vi "Motor-Pega-Vel_Acc.vi"(4 "error out":errorcluster, 7 "MG17Motor in":refnum<k7>) -> (0 "error out 2":errorcluster, 1 "pfAccn":sgl, 2 "pfMaxVel":sgl, 3 "MG17Motor out":refnum<k7>)   [LabVIEW 2014]
doc: "This VI get Velocity and Acceleration of Motor\n\nAndré Romero - 2023\nandretec@ifsc.usp.br\nIFSC - USP"
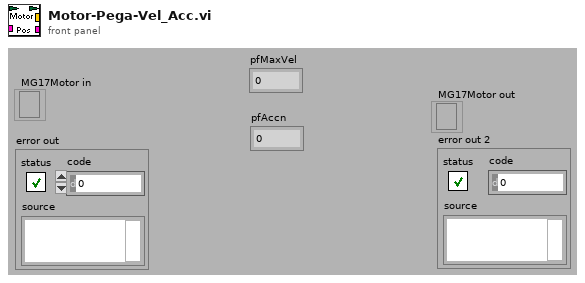
[diagram p1: front panel]
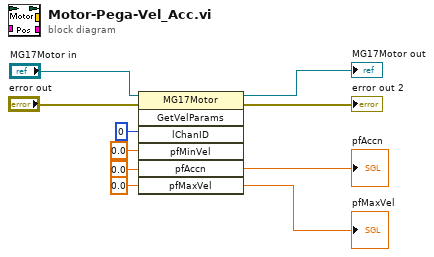
[diagram p0: block diagram]
diagram:
  n1 = invoke class="MG17Motor" method="GetVelParams"(reference="MG17Motor in", error in="error out", "lChanID"=0, "pfMinVel"=sgl 0.0 ("pfPosition"), "pfAccn"=sgl 0.0, "pfMaxVel"=sgl 0.0) -> (reference out=→"MG17Motor out":refnum<k7>, error out=→"error out 2":errorcluster, "pfAccn"=→"pfAccn":sgl, "pfMaxVel"=→"pfMaxVel":sgl)  [unwired: 1 in, 3 out]
